vi "dvp Vi Set Ae Target.vi"(10 "AeTarget":i32, 11 "handle":u32) -> (3 "function return":u32(ring))   [LabVIEW 2018, in "LabViewDVPCamera.lvlib"]
doc: "LabviewDvp2Api dvpStatus dvpViSetAeTarget(dvpHandle handle, dvpInt32 AeTarget);"
uses:
  LabViewDVPCamera.lvlib
  LabViewDVPCamera/LabViewDVPCamera.dll
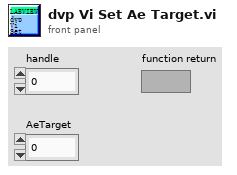
[diagram p1: front panel]
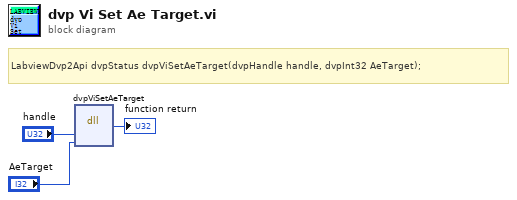
[diagram p0: block diagram]
diagram:
  # "LabviewDvp2Api dvpStatus dvpViSetAeTarget(dvpHandle handle, dvpInt32 AeTarget);"
  n1 = dll-call lib="C:/Program Files (x86)/DVP2 Labview cn 64/Sample/LabViewDVPCamera/LabViewDVPCamera.*" fn="dvpViSetAeTarget"("handle"="handle", "AeTarget"="AeTarget") -> (→"function return":u32)  [unwired: 5 in, 2 out]
